vi "Configure Voltage.vi"(8 "error in (no error)":errorcluster, 10 "Voltage":dbl, 11 "E364x in":refnum<class "E364x.lvclass">) -> (0 "error out":errorcluster, 3 "E364x out":refnum<class "E364x.lvclass">)   [LabVIEW 2020, in "E364x.lvclass"]
uses:
  E364x.lvclass
  C:/Sandbox/Git_Sandbox/WiSpry Test Framework source code (LV20)/WiSpry Test Framework/Instruments/Instrument.lvclass
  C:/Sandbox/Git_Sandbox/WiSpry Test Framework source code (LV20)/WiSpry Test Framework/Instruments/Power Supply/Power Supply.lvclass
  Instrument.lvclass/Instrument.ctl
  Power Supply.lvclass/Power Supply.ctl
  Instrument.lvclass
  <instrlib>/Agilent E364X Series/Agilent E364X Series.lvlib
  Power Supply.lvclass
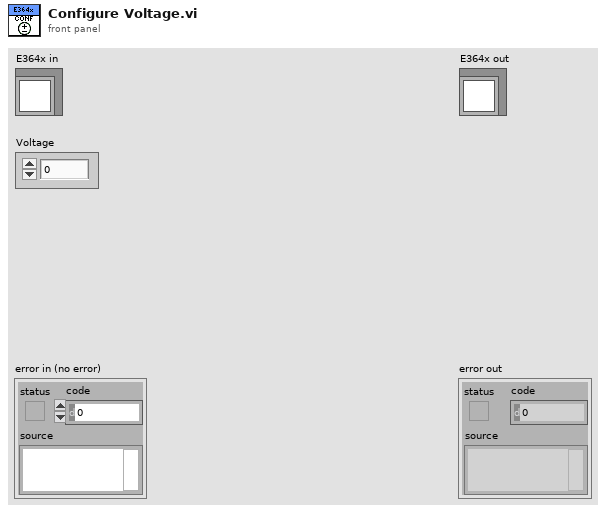
[diagram p1: front panel]
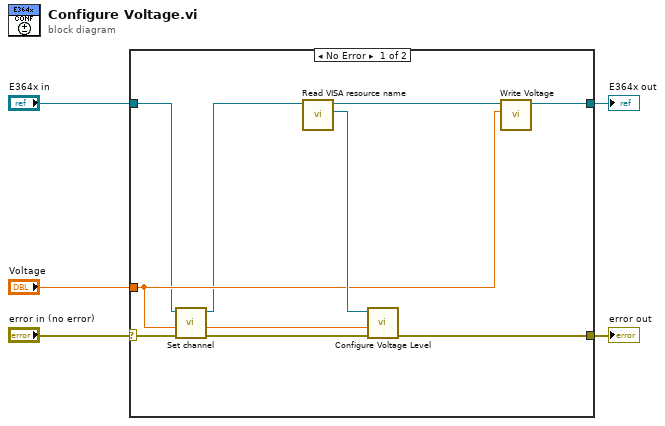
[diagram p0: block diagram]
diagram:
  n1 = case shown="No Error" "error in (no error)" {
    selector: "error in (no error)" -> [w9 w15]
    tunnel: [w12 w16] -> w4
    tunnel: "E364x in" -> [w7 w16]
    tunnel: [w14 w15] -> w2
    tunnel: "Voltage" -> [w10 _]
    frame No Error {
      n2 = call "Set channel.vi"("error in (no error)"=w9, "E364x in"=w7) -> ("error out"=w8:errorcluster, "E364x out"=w6:refnum<class "E364x.lvclass">)  [unwired: 7 in, 1 out]
      n3 = call "Read VISA resource name.vi"("Instrument in"=w6) -> ("VISA resource name"=w13:refnum<visa-resource-name>, "Instrument out"=w11:refnum<class "E364x.lvclass">)  [unwired: 9 in]
      n4 = call <instrlib>:"Configure Voltage Level.vi"("error in (no error)"=w8, "Level (0.0 Volts)"=w10, "VISA resource name"=w13) -> ("error out"=w14:errorcluster)  [unwired: 7 in, 1 out]
      n5 = call "Write Voltage.vi"("Voltage"=w10, "Power Supply in"=w11) -> ("Power Supply out"=w12:refnum<class "E364x.lvclass">)  [unwired: 9 in]
    }
    frame Error {
    }
  }
  "error out" <- w2
  "E364x out" <- w4
